vi "read_IMU Main_TDMS.vi"() -> ()   [LabVIEW 2013]
uses:
  IMU_Data_Type_Def.ctl
  <vilib>/Platform/TimedLoop/XDataNode/timing_clust.ctl
  <vilib>/Platform/TimedLoop/XDataNode/nitl_modes.ctl
  <vilib>/Platform/TimedLoop/XDataNode/wakeup.ctl
  <vilib>/platform/TimedLoop/XDataNode/XDataNode.xnode
  <vilib>/Platform/TimedLoop/XDataNode/XDNodeRunTimeDep.lvlib
panel:
  in  "Period (sampling) [ms]":i64=10
  in  "TDMS: file name":string caption="default name"
  in  "channel name(s)":string[](array[string])
  in  "group name":string
  in  "error in":errorcluster
  out "appended array":dbl[](array[numeric])
  out "Less then desired frequency":bool
  out "IMU_Data_simple":T1
  in  "Stop Button":bool
  out "error out":errorcluster
  out "TDMS: File path":path caption="Filename Out"
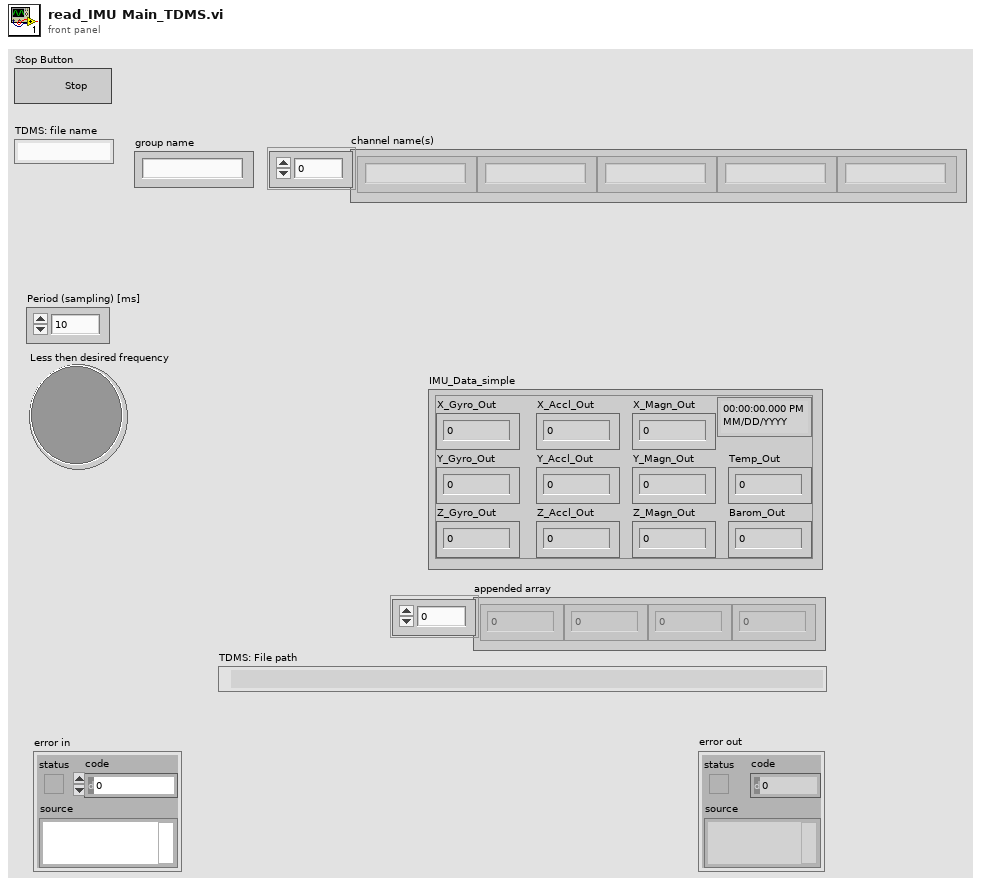
[diagram p1: front panel]
types:
  T1 = typedef "IMU_Data_Type_Def.ctl" = cluster{timestamp, "X_Gyro_Out":dbl, "Y_Gyro_Out":dbl, "Z_Gyro_Out":dbl, "X_Accl_Out":dbl, "Y_Accl_Out":dbl, "Z_Accl_Out":dbl, "X_Magn_Out":dbl, "Y_Magn_Out":dbl, "Z_Magn_Out":dbl, "Temp_Out":dbl, "Barom_Out":dbl}
  T2 = enum16{"open", "open or create", "create or replace", "create", "open (read-only)"}
  T3 = typedef "XDNodeRunTimeDep.lvlib/timing_clust.ctl" = cluster{"Expected End [f-1]":u64, "Actual End [f-1]":u64, "Finished Late? [f-1]":bool, "Expected End [i-1]":u64, "Actual End [i-1]":u64, "Finished Late? [i-1]":bool, "Expected Start [i]":u64, "Actual Start [i]":u64, "Expected Start [f]":u64, "Actual Start [f]":u64, "Source Name":string, "Structure Name":string, "Period":i64, "Deadline":i64, "Offset":i64, "Start":i64, "Priority":i32, "Timeout":i32, "Mode":T4, "Wakeup Reason":T5, "Error":errorcluster, "Source Type":string, "Secondary Source Type":string, "Global End Time":u64, "Global Start Time":u64, "Frame Duration":u64, "Iteration Duration":u64, "Assigned CPU":i32, "I/O Scan Engine Mode":u32}
  T4 = typedef "XDNodeRunTimeDep.lvlib/nitl_modes.ctl" = enum32{"No Change", "Process missed periods, maintain original phase", "Discard missed periods, maintain original phase", "Process missed periods, ignore original phase", "Discard missed periods, ignore original phase"}
  T5 = typedef "XDNodeRunTimeDep.lvlib/wakeup.ctl" = enum32{"Normal", "Aborted", "Asynchronous wakeup", "Timing source error", "Timed loop error", "Timeout"}
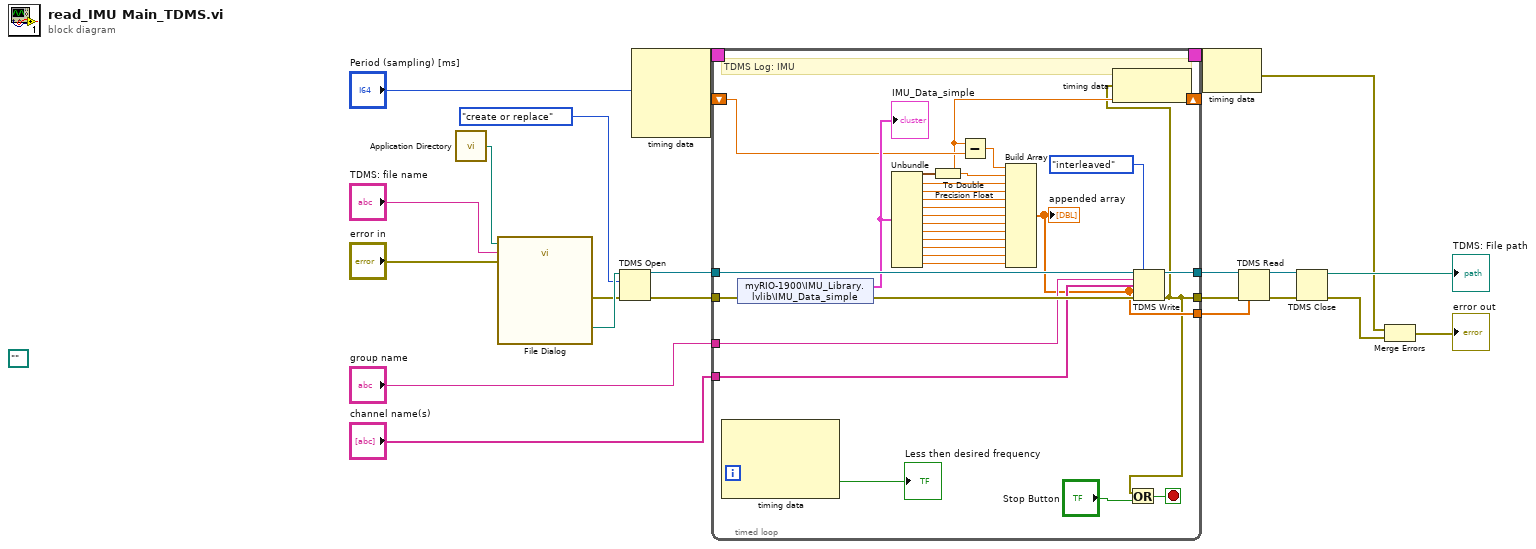
[diagram p0: block diagram]
diagram:
  (unwired) path "" ("Filename Out")
  n1 = call <vilib>:"Application Directory.vi"() -> ("Application Directory"=w22:path)
  n2 = call "File Dialog"("start path"=w22, "default name"="TDMS: file name", "error in"="error in") -> ("selected path"=w20:path, "error out"=w12:errorcluster)  [unwired: 9 in, 2 out]
  n3 = TDMS Open(8:w12, 10:T2."create or replace" ("operation (0:open)"), 11:w20) -> (0:w11:errorcluster, 3:w18:refnum<k34>)  [unwired: 4 in]
  n4 = node-c288("Period (sampling) [ms]") -> (w6:T3)  [unwired: 3 in]
  n5 = timed-loop {
    tunnel: w11 -> [w48]
    tunnel: [w23] -> w15
    shift-right: [w37] -> _
    shift-left: _ -> [w42]
    tunnel: w18 -> [w47]
    tunnel: [w43] -> w17
    tunnel: "channel name(s)" -> [w40]
    tunnel: "group name" -> [w39]
    tunnel: [w25] -> w9
    timing: w6 -> [_]
    timing-out: [_] -> w5
    stop <- w49 stop-if-true
    # "TDMS Log: IMU"
    n6 = node-c288() -> (→"Less then desired frequency":bool)  [unwired: 1 in, 3 out]
    n7 = shared-variable "myRIO-1900\\IMU_Library.lvlib\\IMU_Data_simple"(error in=w48) -> (w46:T1, error out=w45:errorcluster)
    "IMU_Data_simple" <- w46
    n8 = Unbundle(w46) -> (w44:timestamp, "X_Gyro_Out"=w36:dbl, "Y_Gyro_Out"=w35:dbl, "Z_Gyro_Out"=w34:dbl, "X_Accl_Out"=w33:dbl, "Y_Accl_Out"=w31:dbl, "Z_Accl_Out"=w32:dbl, "X_Magn_Out"=w30:dbl, "Y_Magn_Out"=w29:dbl, "Z_Magn_Out"=w28:dbl, "Temp_Out"=w27:dbl, "Barom_Out"=w26:dbl)
    n9 = To Double Precision Float(number=w44) -> (double precision float=w37:dbl)
    n10 = Subtract(x=w37, y=w42) -> (x-y=w38:dbl)
    n11 = Build Array(w38, w37, w36, w35, w34, w33, w31, w32, w30, w29, w28, w27, w26) -> (w25:dbl[])
    "appended array" <- w25
    n12 = TDMS Write(0:w47, 1:enum16{"decimated", "interleaved"}."interleaved" ("data layout (0:decimated)"), 5:w39, 7:w40, 9:w25, 11:w45) -> (4:w43:refnum<k34>, 15:w23:errorcluster)  [unwired: 2 out]
    n13 = node-c288(w23) -> ()  [unwired: 1 out]
    n14 = Or(x=w23, y="Stop Button") -> (x .or. y?=w49:bool)
  }
  n15 = node-c288(w5) -> (w4:errorcluster)
  n16 = TDMS Read(0:w17, 11:w15, 12:w9) -> (4:w16:refnum<k34>, 15:w14:errorcluster)  [unwired: 5 in, 4 out]
  n17 = TDMS Close(8:w14, 11:w16) -> (0:w3:errorcluster, 3:→"TDMS: File path":path)
  n18 = Merge Errors(w4, w3) -> (→"error out":errorcluster)
